vi "CheckScratchAndExit.vi"(11 "Settings":T1={"Name of test"="", "Date"=timestamp(0 s since 1904-01-01), "Location"="", "Template"="", "Soundcard"="", "resolution"=0, "Sampling rate"=0, "Ch1 Gain "=0.0, "Ch2 Gain"=0.0, "Sample time (s)"=0.0, "Pre-trigger (s)"=0.0, "Hammer Threshold"=0.0, "Positions"=0, "Taps/Position"=0, "Set Names"="", "Freq resolution"=0.0, "Hammer cutoff"=0.0, "Mic cutoff"=0.0, "Double bounce "=0.0, "Hammer Cal"=0.0, "dB Offset"=0.0, "Accel Cal"=0.0, "Vibrometer Cal"=0.0, "Mic Cal"=0.0, "Output"=0, "Voltage Cal"=0.0, "Vibrometer Port"="", "Range"=0, "High Pass"=0, "Bandwidth"=0, "X Range"=[], "Y Range"=[], "dB Spread"=0.0, "Trigger"=0, "Ch_1"=0, "Ch_2"=0, "flip?"=FALSE, "60Hz"=FALSE, "Time offset"=0.0, "Piezo Cal"=1.0, "Default Notes"=""} {"Ch_2" min=1 step=1; "Ch_1" min=1 max=100 step=1; "Trigger" items=["Hammer (force)", "Self-tap", "Spacebar"]; "Bandwidth" items=["1 kHz"=1, "5 kHz"=5, "10 kHz"=10, "25 kHz"=25, "50 kHz"=50, "100 kHz"=100]; "High Pass" items=["Off", "13 Hz", "104 Hz"]; "Range" items=["10 mm/s"=1, "20 mm/s"=2, "50 mm/s"=5, "100 mm/s"=10, "200 mm/s"=20, "500 mm/s"=50, "1 m/s"=100, "2 m/s"=200]; "Output" items=["Accelerometer", "Speed (from acceleration)", "Microphone", "Vibrometer", "Piezo"]; "Voltage Cal" format="%#_13g"; "Ch2 Gain" format="%#_13g"; "Ch1 Gain" format="%#_13g"; "Double bounce" min=0.0; "Mic cutoff" min=0.0 format="%#_4g"; "Hammer cutoff" min=0.0 format="%#_4g"; "Freq resolution" min=0.0; "Pre-trigger (s)" format="%#_13g"; "Date" format="%<%H:%M\n%d/%m/%y>T"; "resolution" items=["16 bit"=16, "24 bit"=24, "32 bit"=32]; "Sampling rate" items=["22050 samp/s"=22050, "44100 samp/s"=44100, "48000 samp/s"=48000]}) -> (3 "Ask?":bool)   [LabVIEW 2022 SP3]
uses:
  PreferencesControl.ctl
  Mic/Mic_Global.vi
panel:
  # "Hz"
  # "dB"
  # "dB"
  # "sec"
  # "sec"
  # "mV/Pa"
  # "mV/m/s2"
  # "mV/mm/s"
  # "V/N"
  # "sec"
  # "sec"
  # "mV/N"
  # "a.u."
  # "a.u."
  # "sec"
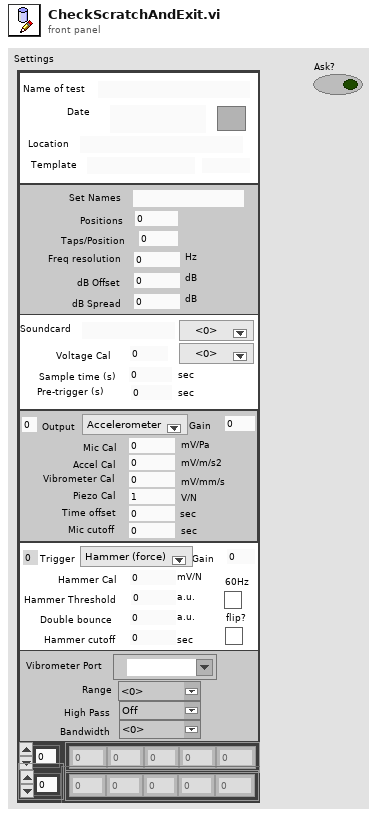
[diagram p1: front panel]
types:
  T1 = typedef "PreferencesControl.ctl" = cluster{"Name of test":string, "Date":timestamp, "Location":string, "Template":string, "Soundcard":string, "resolution":u16, "Sampling rate":u16, "Ch1 Gain ":dbl, "Ch2 Gain":dbl, "Sample time (s)":dbl, "Pre-trigger (s)":dbl, "Hammer Threshold":dbl, "Positions":i16, "Taps/Position":i16, "Set Names":string, "Freq resolution":dbl, "Hammer cutoff":dbl, "Mic cutoff":dbl, "Double bounce ":dbl, "Hammer Cal":dbl, "dB Offset":dbl, "Accel Cal":dbl, "Vibrometer Cal":dbl, "Mic Cal":dbl, "Output":u16, "Voltage Cal":dbl, "Vibrometer Port":refnum<visa-resource-name>, "Range":u16, "High Pass":u16, "Bandwidth":u16, "X Range":cluster{"Minimum":dbl, "Maximum":dbl, "Increment":dbl, "Minor Increment":dbl, "Start":dbl}[], "Y Range":cluster{"Minimum":dbl, "Maximum":dbl, "Increment":dbl, "Minor Increment":dbl, "Start":dbl}[], "dB Spread":dbl, "Trigger":u16, "Ch_1":u8, "Ch_2":u8, "flip?":bool, "60Hz":bool, "Time offset":dbl, "Piezo Cal":dbl, "Default Notes":string}
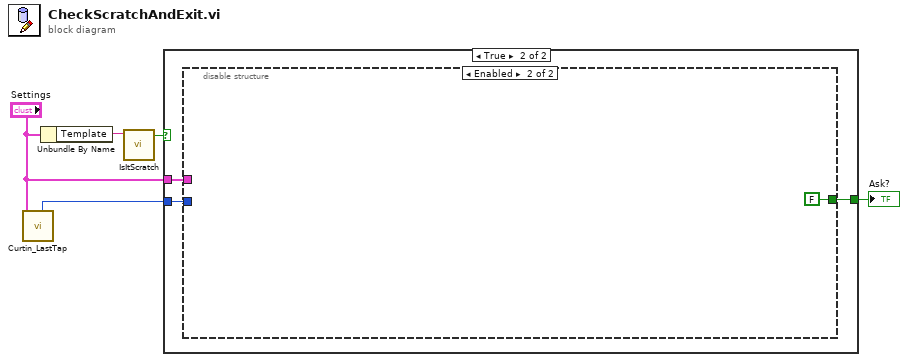
[diagram p0: block diagram]
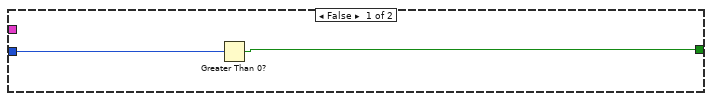
[diagram p2: hidden frame]
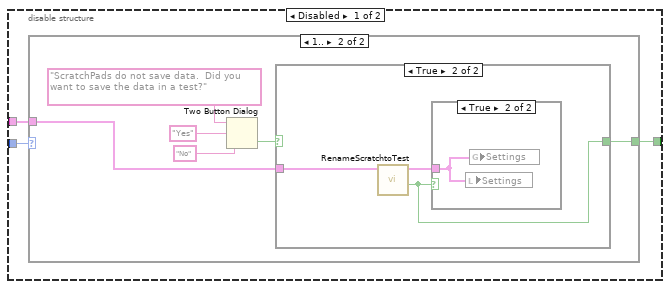
[diagram p3: hidden frame]
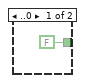
[diagram p4: hidden frame]
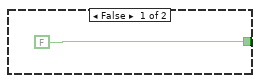
[diagram p5: hidden frame]
diagram:
  n1 = call "Curtin_LastTap.vi"("Settings"="Settings") -> ("files"=w2:i32)  [unwired: 5 in, 5 out]
  n2 = Unbundle By Name("Settings") -> ("Template"=w4:string)
  n3 = call "IsItScratch.vi"("Template"=w4) -> ("ScratchPad?"=w3:bool)  [unwired: 10 in]
  n4 = case shown="True" w3 {
    tunnel: [w7 w10] -> w5
    tunnel: w2 -> [w6 w8]
    tunnel: "Settings" -> [_ w9]
    frame False {
      n5 = Greater Than 0?(x=w6) -> (x > 0?=w7:bool)
    }
    frame True {
      n6 = disable-structure shown="Enabled" {
        disable-tunnel: [w13 FALSE ("Ok?")] -> w10
        disable-tunnel: w9 -> [w12 _]
        disable-tunnel: w8 -> [w11 _]
        frame Disabled {
          n7 = case shown="1.." w11 {
            tunnel: [FALSE ("Ok?") w20] -> w13
            tunnel: w12 -> [_ w17]
            frame ..0 {
            }
            frame 1.. {
              n8 = Two Button Dialog(message="ScratchPads do not save data.  Did you want to save the data in a test?", 1:"No" ("F button name (\"Cancel\")"), 2:"Yes" ("F button name (\"Cancel\")")) -> (T button?=w19:bool)
              n9 = case shown="True" w19 {
                tunnel: [FALSE w22] -> w20
                tunnel: w17 -> [_ w23]
                frame False {
                }
                frame True {
                  n10 = call "RenameScratchtoTest.vi"("Settings"=w23) -> ("Ok?"=w22:bool, "Settings Out"=w24:T1)  [unwired: 8 in, 1 out]
                  n11 = case shown="True" w22 {
                    tunnel: w24 -> [_ w25]
                    frame False {
                    }
                    frame True {
                      n12 = local write "Settings"(w25) -> ()
                      n13 = global write "Mic_Global.vi" "Settings"(w25) -> ()
                    }
                  }
                }
              }
            }
          }
        }
        frame Enabled {
        }
      }
    }
  }
  "Ask?" <- w5
